vi "DMM_DC-RMS Current Meas Configure and Measure.vi"(0 "DMM Handle In":refnum<k15>, 2 "Execution Option":T8, 5 "Function Settings":T2={"Range and Function"=enum."DC Current Auto Range", "Resolution in Digits"=5.5} {"Resolution in Digits" items=["3 1/2"=3.5, "4 1/2"=4.5, "5 1/2"=5.5, "6 1/2"=6.5, "7 1/2"=7.5]}, 7 "Timing & Trigger Settings":T5={"AC Min Frequency (Hz)"=40.0, "Aperture Time (s)"=-1.0, "Settle Time (s)"=-1.0, "Trigger Settings"={"Trigger Delay (sec)"=-1.0, "Enable Trigger?"=FALSE, "Trigger Source"=enum."Immediate", "Slope"=enum."Rising Edge"}} caption="Timing and Trigger Settings" {"Trigger Settings"."Trigger Delay (sec)" format="%.4f"; "AC Min Frequency (Hz)" format="%.2f"}, 11 "error in":errorcluster) -> (4 "DMM Handle Out":refnum<k15>, 6 "Measurement":T1={"Measured Value"=0.0, "Out of Range"=FALSE, "Unit"="A(dc)", "Measurement"="0.0000mA (dc)"} {"Measured Value" format="%^#_9e"}, 8 "DMM Execution Settings":T4={"Absolute\nResolution"=0.0, "Input Resistance\n(Ohm)"=0.0, "Digits\nResolution"=0.0, "Range"=0.0, "Minimum\nFrequency (Hz)"=0.0, "Aperture\nTime (s)"=0.0, "Auto Range\nValue"=0.0, "Settle\nTime (s)"=0.0, "Function"=3} {"Function" items=["DC Volts"=1, "AC Volts"=2, "DC Current"=3, "AC Current"=4, "2-Wire Resistance"=5, "4-Wire Resistance"=101, "Frequency"=104, "Period"=105, "AC Volts DC Coupled"=1001, "Diode"=1002, "Waveform Voltage"=1003, "Waveform Current"=1004, "Capacitance"=1005, "Inductance"=1006, "Temperature"=108]; "Absolute\nResolution" format="%#_6p"; "Input Resistance\n(Ohm)" format="%#_6p"; "Range" format="%#_6p"; "Minimum\nFrequency (Hz)" format="%#_6p"; "Aperture\nTime (s)" format="%#_6p"; "Auto Range\nValue" format="%#_6p"; "Settle\nTime (s)" format="%#_6p"}, 15 "error out":errorcluster)   [LabVIEW 2021, in "DMM_DC-RMS Current Measurement.lvlib"]
doc: "Configures an NI-DMM DC or AC RMS current measurement on the resource provided by the DMM Handle In control according to the given Function, Execution, and Timing & Trigger settings, and then executes the measurement (by default).\n\nAdditionally users can choose to Configure Only without executing the measurement or Measure Only using the existing configuration.."
uses:
  DMM_DC-RMS Current Measurement.lvlib
  Common/Typedefs/Execution Options - Measure.ctl
  Typedefs/Timing & Trigger Settings.ctl
  <instrlib>/niDMM/nidmm.llb/niDMM Trigger.ctl
  <instrlib>/niDMM/nidmm.llb/niDMM Slope.ctl
  Typedefs/DMM Execution Settings.ctl
  Typedefs/Function Settings.ctl
  <instrlib>/niDMM/nidmm.llb/niDMM Resolution in Digits.ctl
  Typedefs/Measurement.ctl
  <instrlib>/niDMM/nidmm.llb/niDMM Configure Measurement Digits.vi
panel:
  # "Inputs"
  # "Outputs"
  # "Execution Settings"
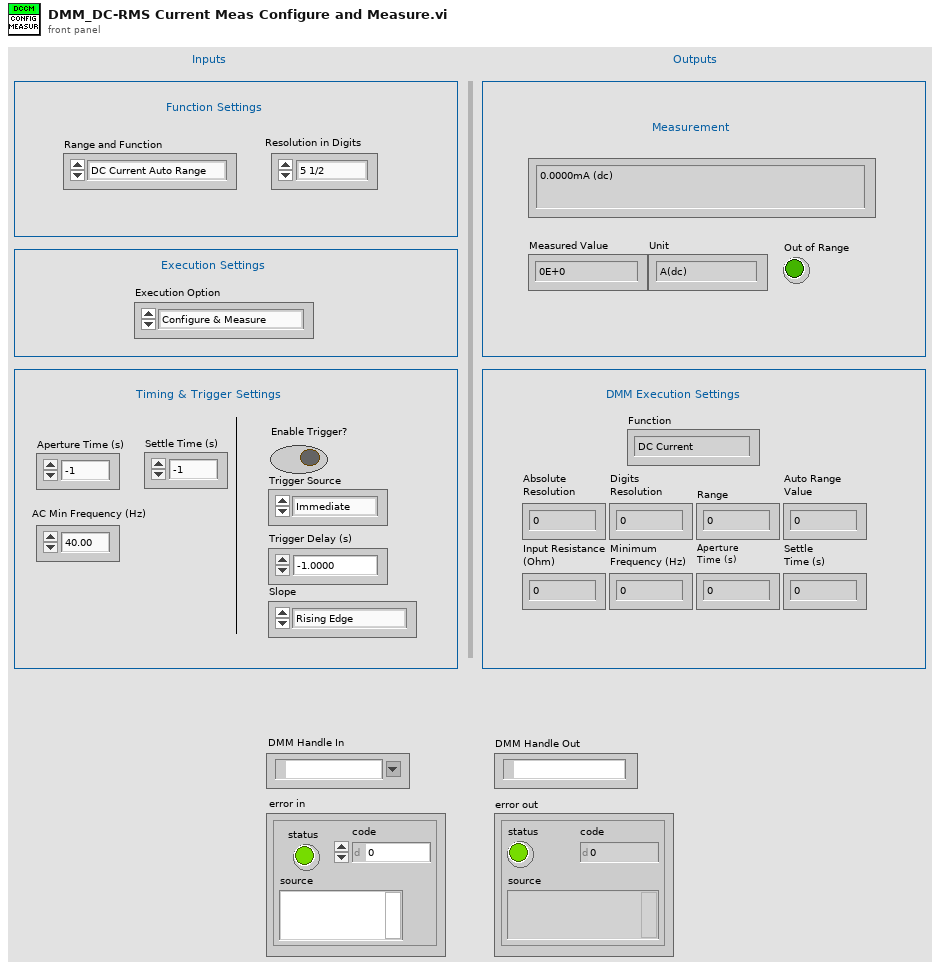
[diagram p1: front panel]
types:
  T1 = typedef "DMM_DC-RMS Current Measurement.lvlib/Measurement.ctl" = cluster{"Measured Value":dbl, "Out of Range":bool, "Unit":string, "Measurement":string}
  T2 = typedef "DMM_DC-RMS Current Measurement.lvlib/Function Settings.ctl" = cluster{"Range and Function":enum16{"DC Current Auto Range", "DC 1 uA", "DC 10 uA", "DC 100 uA", "DC 1 mA", "DC 10 mA", "DC 20 mA", "DC 100 mA", "DC 200 mA", "DC 1 A", "DC 3 A", "   ", "AC Current Auto Range", "AC 100 uA", "AC 1 mA", "AC 10 mA", "AC 100 mA", "AC 500 mA", "AC 1 A", "AC 3 A"}, "Resolution in Digits":T3}
  T3 = typedef "niDMM Resolution in Digits.ctl" = dbl
  T4 = typedef "DMM_DC-RMS Current Measurement.lvlib/DMM Execution Settings.ctl" = cluster{"Absolute\nResolution":dbl, "Input Resistance\n(Ohm)":dbl, "Digits\nResolution":dbl, "Range":dbl, "Minimum\nFrequency (Hz)":dbl, "Aperture\nTime (s)":dbl, "Auto Range\nValue":dbl, "Settle\nTime (s)":dbl, "Function":i32}
  T5 = typedef "DMM_DC-RMS Current Measurement.lvlib/Timing & Trigger Settings.ctl" = cluster{"AC Min Frequency (Hz)":dbl, "Aperture Time (s)":dbl, "Settle Time (s)":dbl, "Trigger Settings":cluster{"Trigger Delay (sec)":dbl, "Enable Trigger?":bool, "Trigger Source":T6, "Slope":T7}}
  T6 = typedef "niDMM Trigger.ctl" = enum16{"Immediate", "External", "TTL 0", "TTL 1", "TTL 2", "TTL 3", "TTL 4", "TTL 5", "TTL 6", "Software", "TTL 7", "PXI Star", "LBR Trig 1", "Aux Trig 1"}
  T7 = typedef "niDMM Slope.ctl" = enum16{"Rising Edge", "Falling Edge"}
  T8 = typedef "Execution Options - Measure.ctl" = enum16{"Configure & Measure", "Configure only", "Measure only"}
  T9 = typedef "niDMM Function.ctl" = enum16{"DC Volts", "AC Volts", "DC Current", "AC Current", "2-wire Resistance", "4-wire Resistance", "Diode", "Frequency", "Period", "AC Volts DC Coupled", "Capacitance", "Inductance", "Temperature"}
  T10 = cluster{"Range":dbl, "Function":T9, "Freq_Period AC Range":dbl, "Resolution in Digits":T3}
  T11 = cluster{"Trigger Delay (sec)":dbl, "Enable Trigger?":bool, "Trigger Source":T6, "Slope":T7}
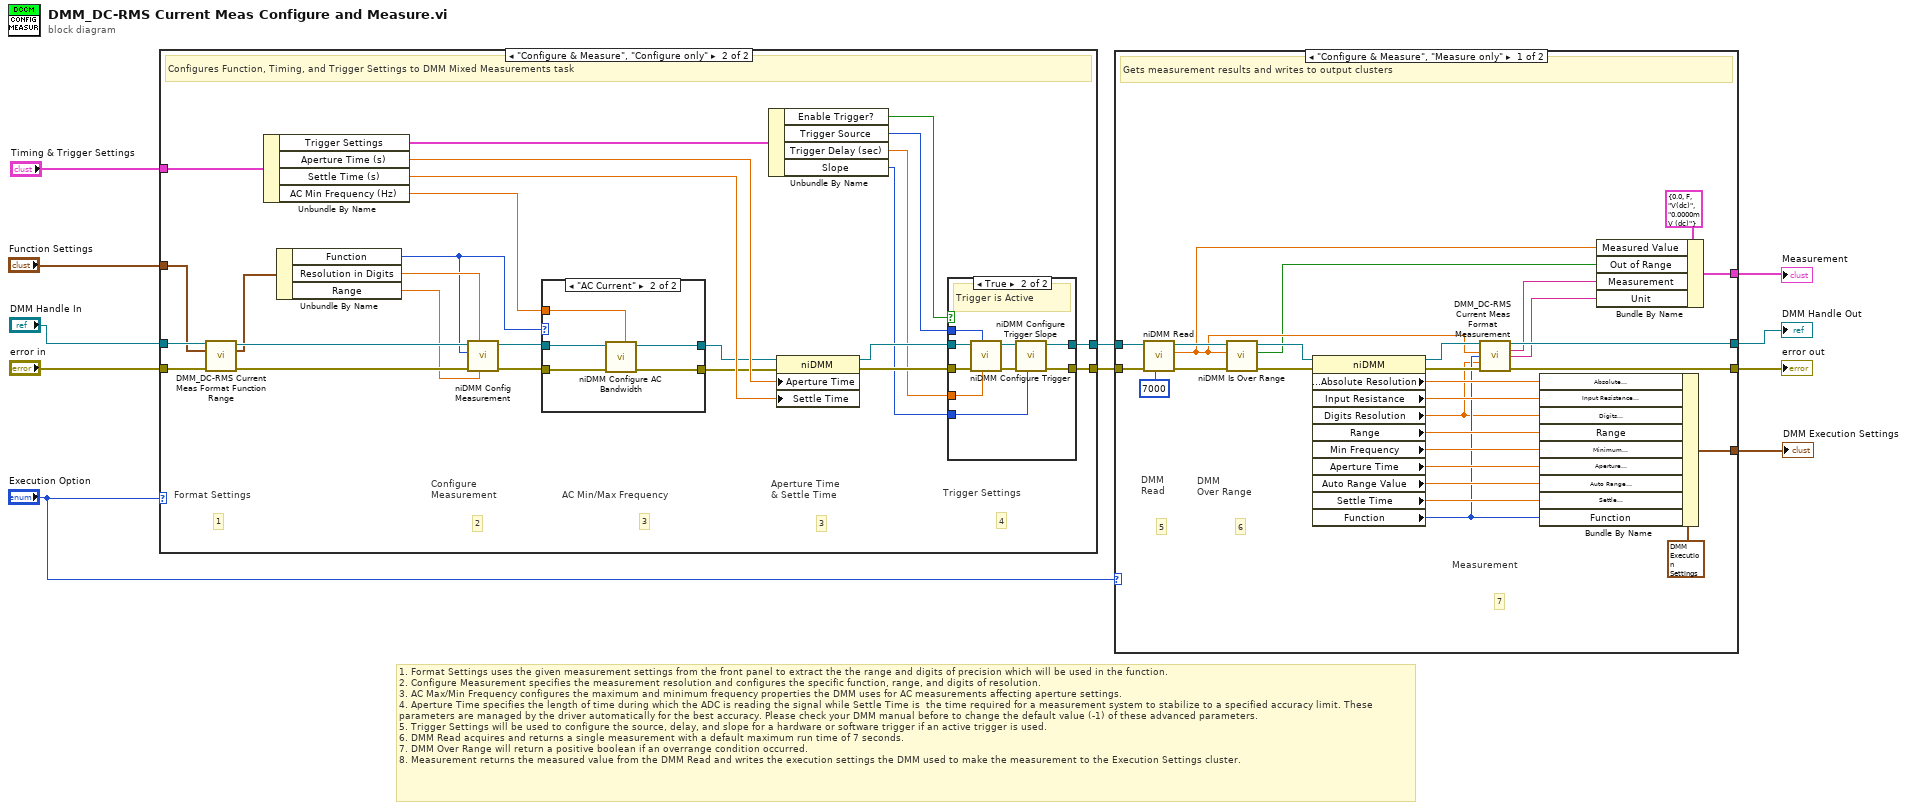
[diagram p0: block diagram]
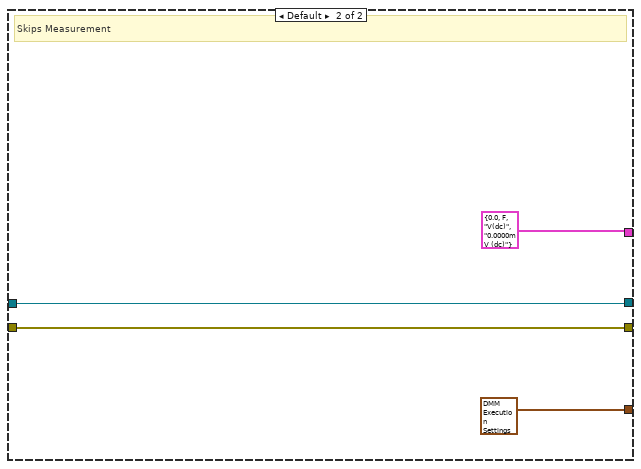
[diagram p2: hidden frame]
diagram:
  # "1. Format Settings uses the given measurement settings from the front panel to extract the the range and digits of precision which will be used in the function.\n2. Configure Measurement specifies the measurement resolution and configures the specific function, range, and digits of resolution.\n3. AC Max/Min Frequency configures the maximum and minimum frequency properties the DMM uses for AC measurements affecting aperture settings.\n4. Aperture Time specifies the length of time during which the ADC is reading the signal while Settle Time is  the time required for a measurement system to stabilize to a specified accuracy limit. These parameters are managed by the driver automatically for the best accuracy. Please check your DMM manual before to change the default value (-1) of these advanced parameters.\n5. Trigger Settings will be used to configure the source, delay, and slope for a hardware or software trigger if an active trigger is used.\n6. DMM Read acquires and returns a single measurement with a default maximum run time of 7 seconds.\n7. DMM Over Range will return a positive boolean if an overrange condition occurred.\n8. Measurement returns the measured value from the DMM Read and writes the execution settings the DMM used to make the measurement to the Execution Settings cluster."
  n1 = case shown="\"Configure & Measure\", \"Configure only\"" "Execution Option" {
    tunnel: [w13 w37] -> w11
    tunnel: [w12 w36] -> w10
    tunnel: "Timing & Trigger Settings" -> [_ w35]
    tunnel: "DMM Handle In" -> [w13 w26]
    tunnel: "Function Settings" -> [_ w22]
    tunnel: "error in" -> [w12 w24]
    frame "Measure only" {
      # "Skips Configurations (Function, Timing and Trigger Settings)"
    }
    frame "Configure & Measure", "Configure only" {
      # "3"
      # "AC Min/Max Frequency"
      # "3"
      # "Aperture Time \n& Settle Time"
      # "1"
      # "Format Settings"
      # "4"
      # "2"
      # "Configure\nMeasurement"
      # "Trigger Settings"
      # "Configures Function, Timing, and Trigger Settings to DMM Mixed Measurements task"
      n2 = call "DMM_DC-RMS Current Meas Format Function Range.vi"("DMM Handle In"=w26, "Function Settings In"=w22, "error in"=w24) -> ("DMM Handle Out"=w25:refnum<k15>, "Function Settings Out"=w23:T10, "error out"=w27:errorcluster)  [unwired: 10 in]
      n3 = Unbundle By Name(w35) -> ("Trigger Settings"=w31:T11, "Aperture Time (s)"=w29:dbl, "Settle Time (s)"=w28:dbl, "AC Min Frequency (Hz)"=w17:dbl)
      n4 = Unbundle By Name(w23) -> ("Function"=w15:T9, "Resolution in Digits"=w16:T3, "Range"=w14:dbl)
      n5 = call-poly <instrlib>:"niDMM Config Measurement.vi"("Range"=w14, "Resolution in Digits"=w16, "error in (no error)"=w27, "Function"=w15, "instrument handle"=w25) -> ("error out"=w21:errorcluster, "instrument handle out"=w20:refnum<k15>)  [unwired: 5 in]
      n6 = case shown="\"AC Current\"" w15 {
        tunnel: [w41 w46] -> w18
        tunnel: [w40 w45] -> w19
        tunnel: w20 -> [w41 w44]
        tunnel: w21 -> [w40 w43]
        tunnel: w17 -> [_ w42]
        frame Default {
        }
        frame "AC Current" {
          n7 = call <instrlib>:"niDMM Configure AC Bandwidth.vi"("Min Frequency"=w42, "error in (no error)"=w43, "instrument handle"=w44) -> ("error out"=w45:errorcluster, "instrument handle out"=w46:refnum<k15>)  [unwired: 7 in]
        }
      }
      n8 = Unbundle By Name(w31) -> ("Enable Trigger?"=w34:bool, "Trigger Source"=w33:T6, "Trigger Delay (sec)"=w32:dbl, "Slope"=w30:T7)
      n9 = property class="niDMM"(reference=w18, error in=w19, "Aperture Time"=w29, "Settle Time"=w28) -> (reference out=w38:refnum<k15>, error out=w39:errorcluster)
      n10 = case shown="True" w34 {
        tunnel: w39 -> [w47 w56]
        tunnel: w38 -> [w48 w57]
        tunnel: [w48 w51] -> w37
        tunnel: [w47 w50] -> w36
        tunnel: w33 -> [_ w54]
        tunnel: w32 -> [_ w55]
        tunnel: w30 -> [_ w49]
        frame False {
          # "No Trigger"
        }
        frame True {
          # "Trigger is Active"
          n11 = call <instrlib>:"niDMM Configure Trigger.vi"("Trigger Delay (sec)"=w55, "Trigger Source"=w54, "error in (no error)"=w56, "instrument handle"=w57) -> ("error out"=w53:errorcluster, "instrument handle out"=w52:refnum<k15>)  [unwired: 6 in]
          n12 = call <instrlib>:"niDMM Configure Trigger Slope.vi"("Slope"=w49, "error in (no error)"=w53, "instrument handle"=w52) -> ("error out"=w50:errorcluster, "instrument handle out"=w51:refnum<k15>)  [unwired: 7 in]
        }
      }
    }
  }
  n13 = case shown="\"Configure & Measure\", \"Measure only\"" "Execution Option" {
    tunnel: w11 -> [w85 w88]
    tunnel: w10 -> [w84 w89]
    tunnel: [w68 w88] -> w6
    tunnel: [w67 w89] -> w9
    tunnel: [w59 T4 {"Absolute\nResolution"=0.0, "Input Resistance\n(Ohm)"=0.0, "Digits\nResolution"=0.0, "Range"=0.0, "Minimum\nFrequency (Hz)"=0.0, "Aperture\nTime (s)"=0.0, "Auto Range\nValue"=0.0, "Settle\nTime (s)"=0.0, "Function"=1} ("Execution Settings 2")] -> w3
    tunnel: [w73 T1 {"Measured Value"=0.0, "Out of Range"=FALSE, "Unit"="V(dc)", "Measurement"="0.0000mV (dc)"}] -> w1
    frame "Configure & Measure", "Measure only" {
      # "6"
      # "DMM \nOver Range"
      # "5"
      # "DMM \nRead"
      # "7"
      # "Measurement"
      # "Gets measurement results and writes to output clusters"
      n14 = call <instrlib>:"niDMM Read.vi"("Maximum Time (msec)"=7000, "error in (no error)"=w84, "instrument handle"=w85) -> ("error out"=w82:errorcluster, "Measurement"=w62:dbl, "instrument handle out"=w83:refnum<k15>)  [unwired: 6 in]
      n15 = call <instrlib>:"niDMM Is Over Range.vi"("error in (no error)"=w82, "Measurement"=w62, "instrument handle"=w83) -> ("error out"=w80:errorcluster, "Over Range?"=w61:bool, "instrument handle out"=w81:refnum<k15>)  [unwired: 6 in]
      n16 = property class="niDMM"(reference=w81, error in=w80) -> (reference out=w70:refnum<k15>, error out=w69:errorcluster, "Configuration:Absolute Resolution"=w72:dbl, "Input Resistance"=w79:dbl, "Digits Resolution"=w63:dbl, "Range"=w78:dbl, "Min Frequency"=w77:dbl, "Aperture Time"=w76:dbl, "Auto Range Value"=w75:dbl, "Settle Time"=w74:dbl, "Function"=w64:i32)
      n17 = call "DMM_DC-RMS Current Meas Format Measurement.vi"("DMM Handle In"=w70, "Measured Value"=w62, "Function"=w64, "Digits Resolution"=w63, "error in"=w69) -> ("DMM Handle Out"=w68:refnum<k15>, "Measurement"=w66:string, "Unit"=w65:string, "error out"=w67:errorcluster)  [unwired: 7 in]
      n18 = Bundle By Name(cluster=T4 {"Absolute\nResolution"=0.0, "Input Resistance\n(Ohm)"=0.0, "Digits\nResolution"=0.0, "Range"=0.0, "Minimum\nFrequency (Hz)"=0.0, "Aperture\nTime (s)"=0.0, "Auto Range\nValue"=0.0, "Settle\nTime (s)"=0.0, "Function"=1} ("Execution Settings"), "Absolute\nResolution"=w72, "Input Resistance\n(Ohm)"=w79, "Digits\nResolution"=w63, "Range"=w78, "Minimum\nFrequency (Hz)"=w77, "Aperture\nTime (s)"=w76, "Auto Range\nValue"=w75, "Settle\nTime (s)"=w74, "Function"=w64) -> (w59:T4)
      n19 = Bundle By Name(cluster=T1 {"Measured Value"=0.0, "Out of Range"=FALSE, "Unit"="V(dc)", "Measurement"="0.0000mV (dc)"}, "Measured Value"=w62, "Out of Range"=w61, "Measurement"=w66, "Unit"=w65) -> (w73:T1)
    }
    frame Default {
      # "Skips Measurement"
    }
  }
  "error out" <- w9
  "DMM Handle Out" <- w6
  "DMM Execution Settings" <- w3
  "Measurement" <- w1
